vi "VFH-read_file-Excel.vi"(8 "error in (no error)":errorcluster, 10 "file path (dialog if empty)":path=path "C:/projects/UNI/VNA/Jorgmalinger20240615/vann0.01M-20240625-505.xlsx") -> (0 "error out":errorcluster, 2 "output cluster":T1)   [LabVIEW 2020, in "VFH-VNA_File_Handler.lvlib"]
uses:
  VFH-VNA_File_Handler.lvlib
  <vilib>/Utility/NIReport.llb/NI_report.lvclass
  VFH-file_cluster-Expensive.ctl
  <vilib>/addons/_office/excel.llb/Excel Get Data ([dbl]).vi
panel:
  out "Waveform Graph":dbl[](graph)
  out "Output":dbl[][](array[numeric])
  out "Sheet 1 Data":dbl[][](array[numeric]) format="%.2f"
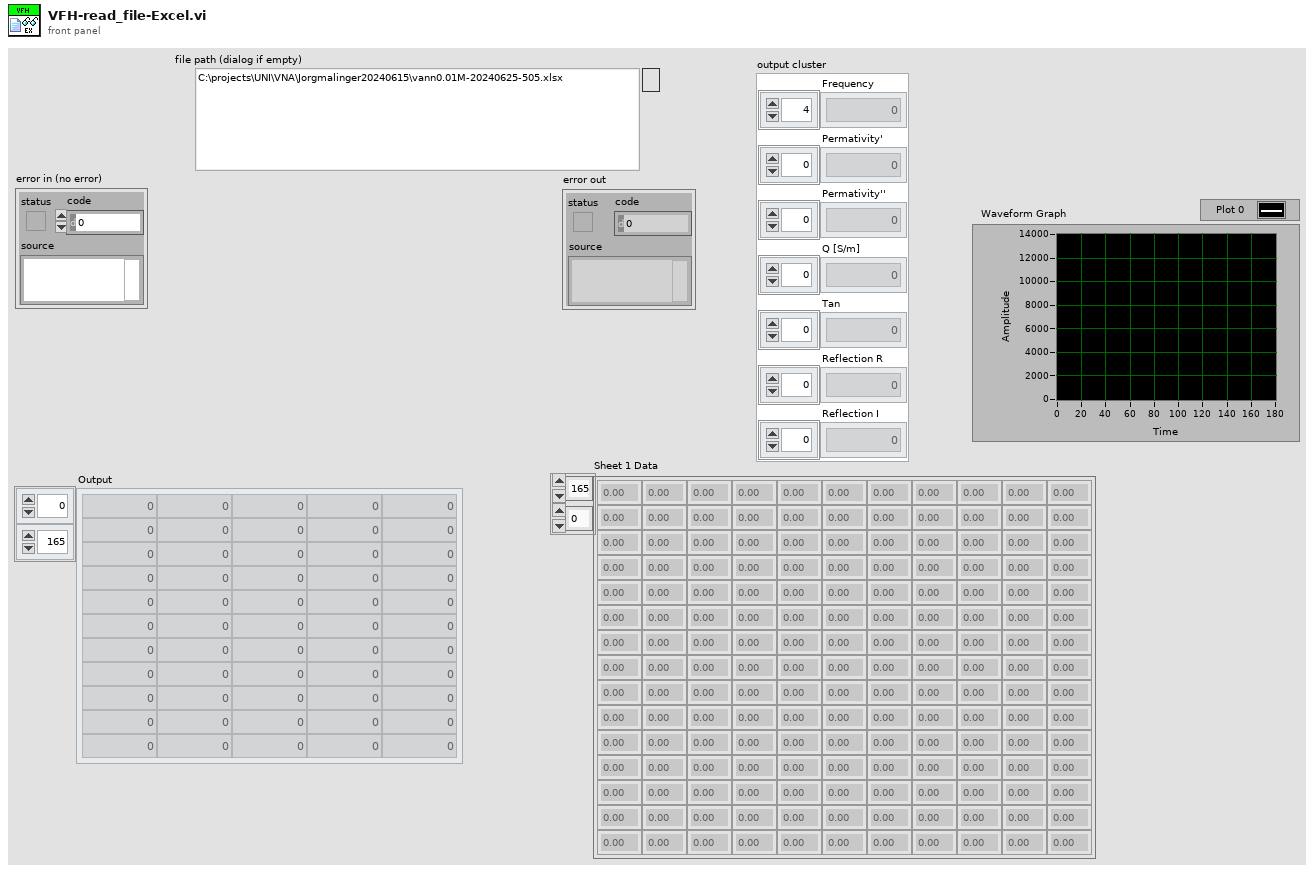
[diagram p1: front panel]
types:
  T1 = typedef "VFH-VNA_File_Handler.lvlib/VFH-file_cluster-Expensive.ctl" = cluster{"Frequency":dbl[], "Permativity'":dbl[], "Permativity''":dbl[], "Q [S/m]":dbl[], "Tan":dbl[], "Reflection R":dbl[], "Reflection I":dbl[]}
  T2 = enum16{"Standard Report", "HTML", "Word", "Excel"}
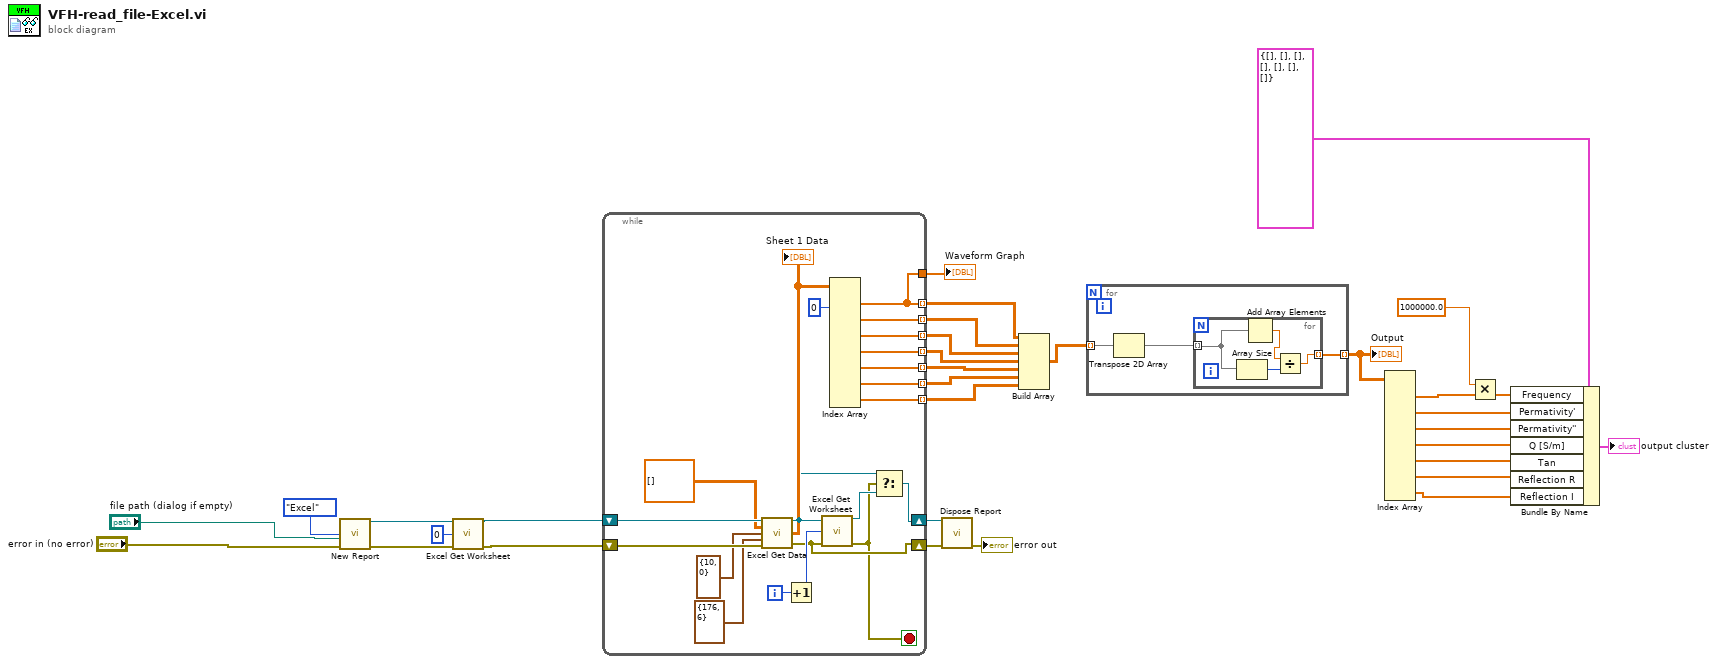
[diagram p0: block diagram]
diagram:
  n1 = call <vilib>:"New Report.vi"("report type"=T2."Excel", "template (empty)"="file path (dialog if empty)", "error in (no error)"="error in (no error)") -> ("report out"=w8:refnum<class "NI_report.lvclass">, "error out"=w7:errorcluster)  [unwired: 3 in, 8 out]
  n2 = call <vilib>:"Excel Get Worksheet.vi"("report in"=w8, "worksheet index (0)"=0, "error in (no error)"=w7) -> ("report out"=w5:refnum<class "NI_report.lvclass">, "error out"=w4:errorcluster)  [unwired: 11 out]
  n3 = while {
    shift-right: [w35] -> w31
    shift-left: w5 -> [w53]
    shift-right: [w38] -> w30
    shift-left: w4 -> [w51]
    tunnel: [w33] -> w28 mode=indexing
    tunnel: [w46] -> w27 mode=indexing
    tunnel: [w45] -> w25 mode=indexing
    tunnel: [w44] -> w24 mode=indexing
    tunnel: [w43] -> w23 mode=indexing
    tunnel: [w42] -> w22 mode=indexing
    tunnel: [w41] -> w21 mode=indexing
    tunnel: [w33] -> w1
    i -> [w40]
    stop <- w34 stop-if-true
    n4 = call-poly <vilib>:"Excel Get Data.vi"("report in"=w53, "data type"=dbl[][] [], "start (-1, -1)"=cluster{"row":i32, "column":i32} {"row"=10, "column"=0}, "end (-1, -1)"=cluster{"row":i32, "column":i32} {"row"=176, "column"=6}, "error in (no error)"=w51) -> ("report out"=w37:refnum<class "NI_report.lvclass">, "data"=w47:dbl[][], "error out"=w38:errorcluster)  [unwired: 8 out]
    "Sheet 1 Data" <- w47
    n5 = Increment(x=w40) -> (x+1=w39:i32)
    n6 = call <vilib>:"Excel Get Worksheet.vi"("report in"=w37, "worksheet index (0)"=w39, "error in (no error)"=w38) -> ("report out"=w36:refnum<class "NI_report.lvclass">, "error out"=w34:errorcluster)  [unwired: 11 out]
    n7 = Index Array(array=w47, index (col) #1=0 ("disabled index (col)")) -> (element #1=w33:dbl[], element #2=w46:dbl[], element #3=w45:dbl[], element #4=w44:dbl[], element #5=w43:dbl[], element #6=w42:dbl[], element #7=w41:dbl[])  [unwired: 13 in]
    n8 = Select(t=w37, s=w34, f=w36) -> (s? t:f=w35:refnum<class "NI_report.lvclass">)
  }
  "Waveform Graph" <- w1
  n9 = call-dynamic "Dispose Report.vi"("report in"=w31, "error in (no error)"=w30) -> ("error out"=→"error out":errorcluster)  [unwired: 3 in, 10 out]
  n10 = Build Array(w28, w27, w25, w24, w23, w22, w21) -> (w26:dbl[][][])
  n11 = for {
    tunnel: w26 -> [w54] mode=indexing
    tunnel: [w55] -> w20 mode=indexing
    n12 = Transpose 2D Array(2D array=w54) -> (transposed array=w56:dbl[][])
    n13 = for {
      tunnel: w56 -> [w60] mode=indexing
      tunnel: [w59] -> w55 mode=indexing
      n14 = Array Size(array=w60) -> (size(s)=w57:i32)
      n15 = Add Array Elements(numeric array=w60) -> (sum=w58:dbl)
      n16 = Divide(x=w58, y=w57) -> (x/y=w59:dbl)
    }
  }
  "Output" <- w20
  n17 = Index Array(array=w20) -> (element #1=w19:dbl[], element #2=w18:dbl[], element #3=w17:dbl[], element #4=w16:dbl[], element #5=w15:dbl[], element #6=w14:dbl[], element #7=w13:dbl[])  [unwired: 14 in]
  n18 = Multiply(x=1000000.0 ("Numeric"), y=w19) -> (x*y=w3:dbl[])
  n19 = Bundle By Name(cluster=T1 {"Frequency"=[], "Permativity'"=[], "Permativity''"=[], "Q [S/m]"=[], "Tan"=[], "Reflection R"=[], "Reflection I"=[]} ("output cluster"), "Frequency"=w3, "Permativity'"=w18, "Permativity''"=w17, "Q [S/m]"=w16, "Tan"=w15, "Reflection R"=w14, "Reflection I"=w13) -> (→"output cluster":T1)
